vi "Configure Alarm.vi"(0 "VISA resource name":refnum<visa-resource-name>, 1 "Enable Latch (F: Enable)":bool, 2 "Audible  (F: Off)":bool, 3 "Visible  (F: Off)":bool, 5 "Channel (1:1)":u16(ring)=1 items=["All Channels", "1", "2", "3", "4", "5", "6", "7", "8", "9", "10", "11", "12", "13", "14", "15", "16", "A (Control Input)"], 7 "Enable Alarm  (F: Off)":bool, 11 "error in (no error)":errorcluster, 12 "High Value (0.00000E+0)":dbl min=0.0 max=100000000.0 step=1e-06 format="%^.5e", 13 "Low Value (0.00000E+0)":dbl min=0.0 max=100000000.0 step=1e-06 format="%^.5e", 14 "Deadband (0.00000E+0)":dbl min=0.0 max=100000000.0 step=1e-06 format="%^.5e") -> (4 "VISA resource name out":refnum<visa-resource-name>, 15 "error out":errorcluster)   [LabVIEW 2015, in "Lake Shore 372.lvlib"]
doc: "Configures the 372 alarm functions. Control is provided over the alarm high and low setpoints, trigger inside/outside status, audible alarm status, and alarm active status. A display annunciator and audible beeper signal an active alarm at the instrument."
uses:
  <instrlib>/Lake Shore 372/Lake Shore 372.lvlib
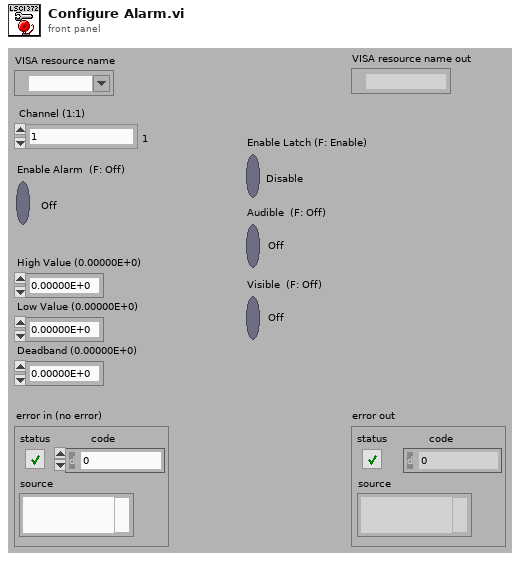
[diagram p1: front panel]
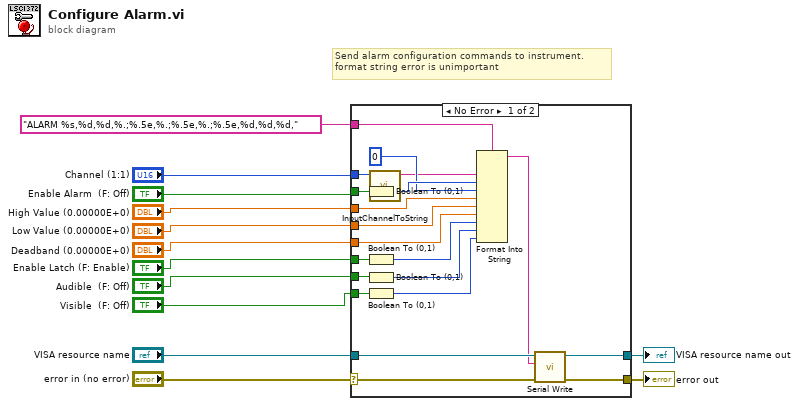
[diagram p0: block diagram]
diagram:
  # "Send alarm configuration commands to instrument.\nformat string error is unimportant"
  n1 = case shown="No Error" "error in (no error)" {
    selector: "error in (no error)" -> [w15 w34]
    tunnel: "VISA resource name" -> [w33 w35]
    tunnel: [w32 w34] -> w12
    tunnel: [w31 w35] -> w11
    tunnel: "ALARM %s,%d,%d,%.;%.5e,%.;%.5e,%.;%.5e,%d,%d,%d," ("format string") -> [w30 _]
    tunnel: "Channel (1:1)" -> [w14 _]
    tunnel: "Enable Alarm  (F: Off)" -> [w22 _]
    tunnel: "High Value (0.00000E+0)" -> [w21 _]
    tunnel: "Low Value (0.00000E+0)" -> [w20 _]
    tunnel: "Deadband (0.00000E+0)" -> [w19 _]
    tunnel: "Enable Latch (F: Enable)" -> [w18 _]
    tunnel: "Audible  (F: Off)" -> [w17 _]
    tunnel: "Visible  (F: Off)" -> [w16 _]
    frame No Error {
      n2 = Boolean To (0,1)(Boolean=w22) -> (0, 1=w29:i16)
      n3 = Boolean To (0,1)(Boolean=w18) -> (0, 1=w27:i16)
      n4 = Boolean To (0,1)(Boolean=w17) -> (0, 1=w26:i16)
      n5 = Boolean To (0,1)(Boolean=w16) -> (0, 1=w25:i16)
      n6 = call <instrlib>:"InputChannelToString.vi"("Channel (1)"=w14) -> ("Channel Str"=w23:string)  [unwired: 10 in]
      n7 = Format Into String(format string=w30, w23, w29, i16 0 ("0, 1"), w21, w20, w19, w27, w26, w25) -> (resulting string=w24:string)  [unwired: 2 in, 1 out]
      n8 = call <instrlib>:"Serial Write.vi"("error in (no error)"=w15, "Write Buffer (\"\")"=w24, "VISA resource name"=w33) -> ("error out"=w32:errorcluster, "VISA resource name out"=w31:refnum<visa-resource-name>)  [unwired: 6 in, 1 out]
    }
    frame Error {
    }
  }
  "error out" <- w12
  "VISA resource name out" <- w11
